vi "DisableEnableStart.vi"() -> (0 "S6AckVisable":bool, 1 "S5AckVisable":bool, 2 "Station6":T1(ring), 3 "Station5":T1(ring))   [LabVIEW 2018, in "GUI3.lvclass"]
uses:
  GUI3.lvclass
panel:
  out "error out":errorcluster
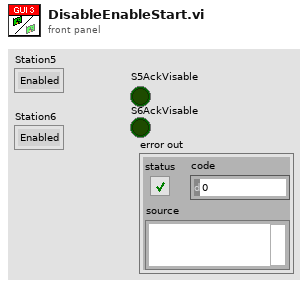
[diagram p1: front panel]
types:
  T1 = enum8{"Enabled", "Disabled", "Disabled and Grayed Out"}
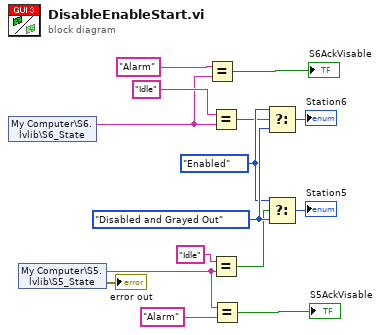
[diagram p0: block diagram]
diagram:
  w14 = T1."Disabled and Grayed Out" ("Disabled")
  w13 = T1."Enabled" ("Disabled")
  n1 = shared-variable "My Computer\\S6.lvlib\\S6_State"() -> (w8:string)  [unwired: 1 in, 1 out]
  n2 = shared-variable "My Computer\\S5.lvlib\\S5_State"() -> (w6:string, error out=→"error out":errorcluster)  [unwired: 1 in]
  n3 = Equal?(x="Alarm" ("y"), y=w8) -> (x = y?=→"S6AckVisable":bool)
  n4 = Equal?(x="Idle" ("y"), y=w8) -> (x = y?=w12:bool)
  n5 = Equal?(x="Idle" ("y"), y=w6) -> (x = y?=w10:bool)
  n6 = Equal?(x=w6, y="Alarm") -> (x = y?=→"S5AckVisable":bool)
  n7 = Select(t=w13, s=w12, f=w14) -> (s? t:f=→"Station6":T1)
  n8 = Select(t=w13, s=w10, f=w14) -> (s? t:f=→"Station5":T1)
